vi "Do Something.vi"(8 "error in (no error)":errorcluster, 10 "Do Something Message":string, 11 "Module ID":i32=-1) -> (0 "error out":errorcluster)   [LabVIEW 2020, in "Client HTTP Post.lvlib"]
doc: "Send the Do something request to the Module's Main.vi.\n_____\nBased on DQMH Project Template 6.0.0.91."
uses:
  Client HTTP Post.lvlib
  Do Something Argument--cluster.ctl
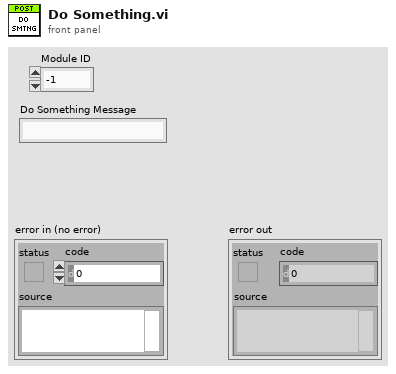
[diagram p1: front panel]
types:
  T1 = typedef "Client HTTP Post.lvlib/Do Something Argument--cluster.ctl" = cluster{"Module ID":i32, "Do Something Msg":string}
  T2 = typedef "Client HTTP Post.lvlib/Request Events--cluster.ctl" = cluster{"Stop Module":refnum<user-event>, "Do Something":refnum<user-event>, "Do Something Else":refnum<user-event>, "Do Something Else and Wait for Reply":refnum<user-event>, "Show Panel":refnum<user-event>, "Hide Panel":refnum<user-event>, "Show Diagram":refnum<user-event>, "Get Module Execution Status":refnum<user-event>}
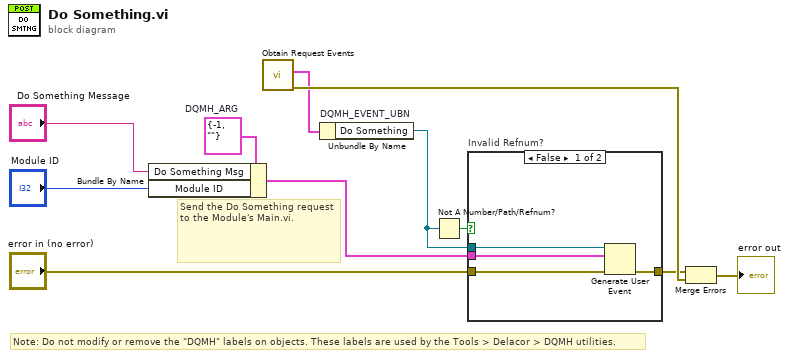
[diagram p0: block diagram]
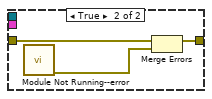
[diagram p2: hidden frame]
diagram:
  w8 = T1 {"Module ID"=-1, "Do Something Msg"=""}  # DQMH_ARG
  # "Note: Do not modify or remove the \"DQMH\" labels on objects. These labels are used by the Tools > Delacor > DQMH utilities."
  # "Send the Do Something request to the Module's Main.vi."
  n1 = Bundle By Name(cluster=w8, "Do Something Msg"="Do Something Message", "Module ID"="Module ID") -> (w3:T1)
  n2 = call "Obtain Request Events.vi"() -> ("error out"=w10:errorcluster, "Client HTTP Post Request Events"=w9:T2)  [unwired: 10 in]
  n3 = Unbundle By Name "DQMH_EVENT_UBN"(w9) -> ("Do Something"=w4:refnum<user-event>)
  n4 = Not A Number/Path/Refnum?(number/path/refnum=w4) -> (NaN/Path/Refnum?=w7:bool)
  n5 = case "Invalid Refnum?" shown="False" w7 {
    tunnel: "error in (no error)" -> [w15 w16]
    tunnel: [w14 w17] -> w6
    tunnel: w3 -> [w13 _]
    tunnel: w4 -> [w12 _]
    frame False {
      n6 = Generate User Event(user event=w12, event data cluster=w13, error in=w15) -> (error out=w14:errorcluster)  [unwired: 1 in, 1 out]
    }
    frame True {
      n7 = call "Module Not Running--error.vi"() -> ("error out"=w18:errorcluster)  [unwired: 11 in]
      n8 = Merge Errors(w16, w18) -> (w17:errorcluster)
    }
  }
  n9 = Merge Errors(w6, w10) -> (→"error out":errorcluster)
